vi "powerdelivery unpack Data Object Attributes.vi"(0 "id":u32, 1 "partner":string, 2 "ruleIndex":string, 5 "result":cluster{"value":i32, "error":i32}, 7 "index":i32, 9 "attributes":u8, 11 "error in (no error)":errorcluster, 12 "powerRole":string) -> (3 "partner out":string, 4 "id out":u32, 6 "result out":cluster{"value":i32, "error":i32}, 8 "ruleIndex out":string, 14 "powerRole out":string, 15 "error out":errorcluster)   [LabVIEW 2014, in "BrainStem2_LabVIEW_Library.lvlib"]
doc: "aLIBEXPORT void __stdcall powerdelivery_unpackDataObjectAttributes ( unsigned int* id, struct Result* result, const int index , const unsigned char attributes , unsigned char * partner , unsigned char * powerRole , unsigned char * ruleIndex ) ;"
uses:
  BrainStem2_LabVIEW_Library.lvlib
  BrainStem2_LabVIEW.dll
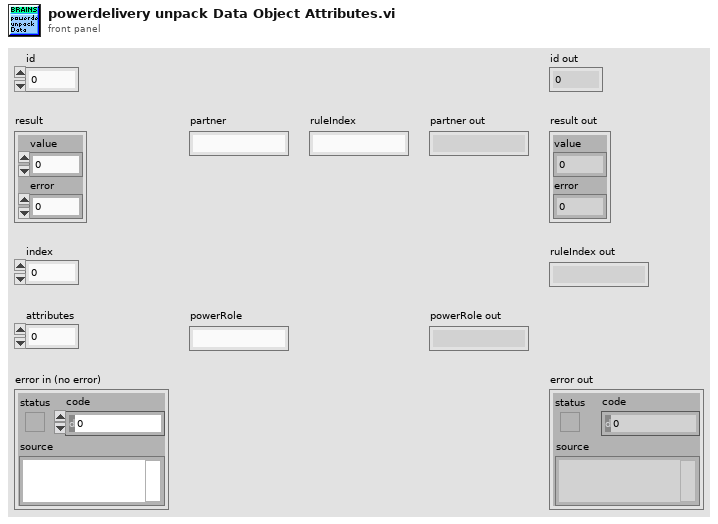
[diagram p1: front panel]
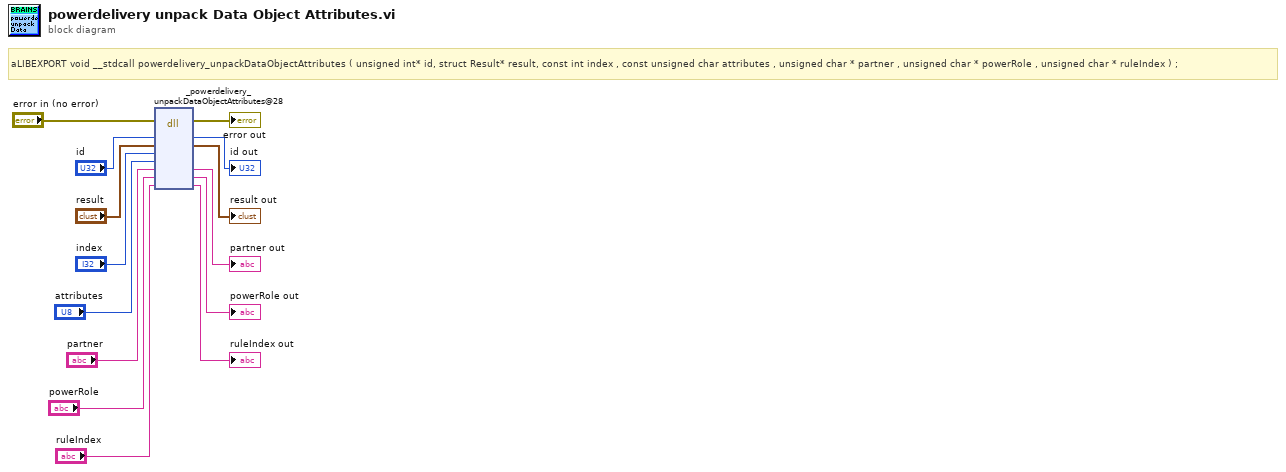
[diagram p0: block diagram]
diagram:
  # "aLIBEXPORT void __stdcall powerdelivery_unpackDataObjectAttributes ( unsigned int* id, struct Result* result, const int index , const unsigned char attributes , unsigned char * partner , unsigned char * powerRole , unsigned char * ruleIndex ) ;"
  n1 = dll-call lib="C:/Users/mitch/Documents/development/acroname/software/acroname/aSource/BrainStem2/BrainStem2_LabVIEW/LabVIEW_2014_Distribution/BrainStem2_LabVIEW_w32/BrainStem2_LabVIEW.*" fn="_powerdelivery_unpackDataObjectAttributes@28"(error in="error in (no error)", "id"="id", "result"="result", "index"="index", "attributes"="attributes", "partner"="partner", "powerRole"="powerRole", "ruleIndex"="ruleIndex") -> (error out=→"error out":errorcluster, "id"=→"id out":u32, "result"=→"result out":cluster{"value":i32, "error":i32}, "partner"=→"partner out":string, "powerRole"=→"powerRole out":string, "ruleIndex"=→"ruleIndex out":string)  [unwired: 5 in, 1 out]
